vi "Turret_Aim.vi"(6 "View Button":bool, 7 "Left Trigger":dbl, 8 "Orange Limit Pressed":bool, 9 "Blue Limit Pressed":bool, 10 "Right Bumper":bool, 11 "Left Bumper":bool) -> ()   [LabVIEW 2020]
uses:
  <vilib>/Rock Robotics/WPI/ThirdParty/Phoenix-LabVIEW/Motor Controller/Controls/CTRE_Phoenix_MotorControl_ControlMode.ctl
  <vilib>/Rock Robotics/WPI/ThirdParty/Phoenix-LabVIEW/Motor Controller/Get/CTRE_Phoenix_MotorController_IntegratedSensorData_TalonFX.vi
  <vilib>/Rock Robotics/Network Tables/NT Read Number.vi
  <vilib>/addons/control/pid/pid.llb/PID (DBL).vi
  <vilib>/Rock Robotics/Network Tables/NT Write Number.vi
  <vilib>/addons/control/pid/NI_PID_pid.lvlib
panel:
  in  "Auto Center PID":T1={"proportional gain (Kc)"=-0.025, "integral time (Ti, min)"=0.0, "derivative time (Td, min)"=2e-05} {"derivative time (Td, min)" format="%.6f"; "integral time (Ti, min)" format="%.3f"; "proportional gain (Kc)" format="%.3f"}
  out "Ty":dbl
  out "Tx":dbl
  in  "Turret Auto Aim PID":T1={"proportional gain (Kc)"=-0.025, "integral time (Ti, min)"=0.0, "derivative time (Td, min)"=2e-05} {"derivative time (Td, min)" format="%.6f"; "integral time (Ti, min)" format="%.3f"; "proportional gain (Kc)" format="%.3f"}
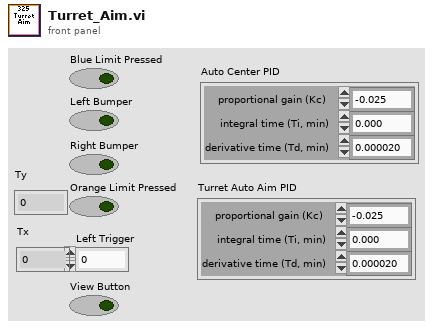
[diagram p1: front panel]
types:
  T1 = cluster{"proportional gain (Kc)":dbl, "integral time (Ti, min)":dbl, "derivative time (Td, min)":dbl}
  T2 = typedef "CTRE_Phoenix_MotorControl_ControlMode.ctl" = u16
  T3 = typedef "WPI_MotorControlDeviceRef.ctl" = cluster{"DeviceStatus":errorcluster, "Type":T4, "PWM":cluster{"PWM Channel":T5, "DeadBand":T6}, "CAN":cluster{"Device Number":u8, "SetOutput VI Ref":variant, "GetOutput VI Ref":variant, "Enable VI Ref":variant, "Disable VI Ref":variant, "Data":variant}, "Invert":bool, "DIO PWM":cluster{"PWM \"Enable\" Channel":T5, "DIOChannel":T7, "PWM Rate":dbl}}
  T4 = typedef "WPI_MotorControlType.ctl" = enum16{"PWM", "CAN", "DIO PWM"}
  T5 = typedef "FPGA_DIOPWMChannel.ctl" = enum8{"PWM 0", "PWM 1", "PWM 2", "PWM 3", "PWM 4", "PWM 5", "PWM 6", "PWM 7", "PWM 8", "PWM 9", "PWM MXP 0", "PWM MXP 1", "PWM MXP 2", "PWM MXP 3", "PWM MXP 4", "PWM MXP 5", "PWM MXP 6", "PWM MXP 7", "PWM MXP 8", "PWM MXP 9", "Invalid"}
  T6 = typedef "WPI_PWMDeadband.ctl" = cluster{"Name":string, "maxPositivePwm":i32, "minPositivePwm":i32, "centerPwm":i32, "maxNegativePwm":i32, "minNegativePwm":i32, "angularRange":u16}
  T7 = typedef "FPGA_DIOChannel.ctl" = enum8{"DIO 0", "DIO 1", "DIO 2", "DIO 3", "DIO 4", "DIO 5", "DIO 6", "DIO 7", "DIO 8", "DIO 9", "DIO MXP 0", "DIO MXP 1", "DIO MXP 2", "DIO MXP 3", "DIO MXP 4", "DIO MXP 5", "DIO MXP 6", "DIO MXP 7", "DIO MXP 8", "DIO MXP 9", "DIO MXP 10", "DIO MXP 11", "DIO MXP 12", "DIO MXP 13", "DIO MXP 14", "DIO MXP 15", "SPI Port CS1", "SPI Port CS2", "SPI Port CS3", "SPI Port MISO", "SPI Port MOSI", "Invalid"}
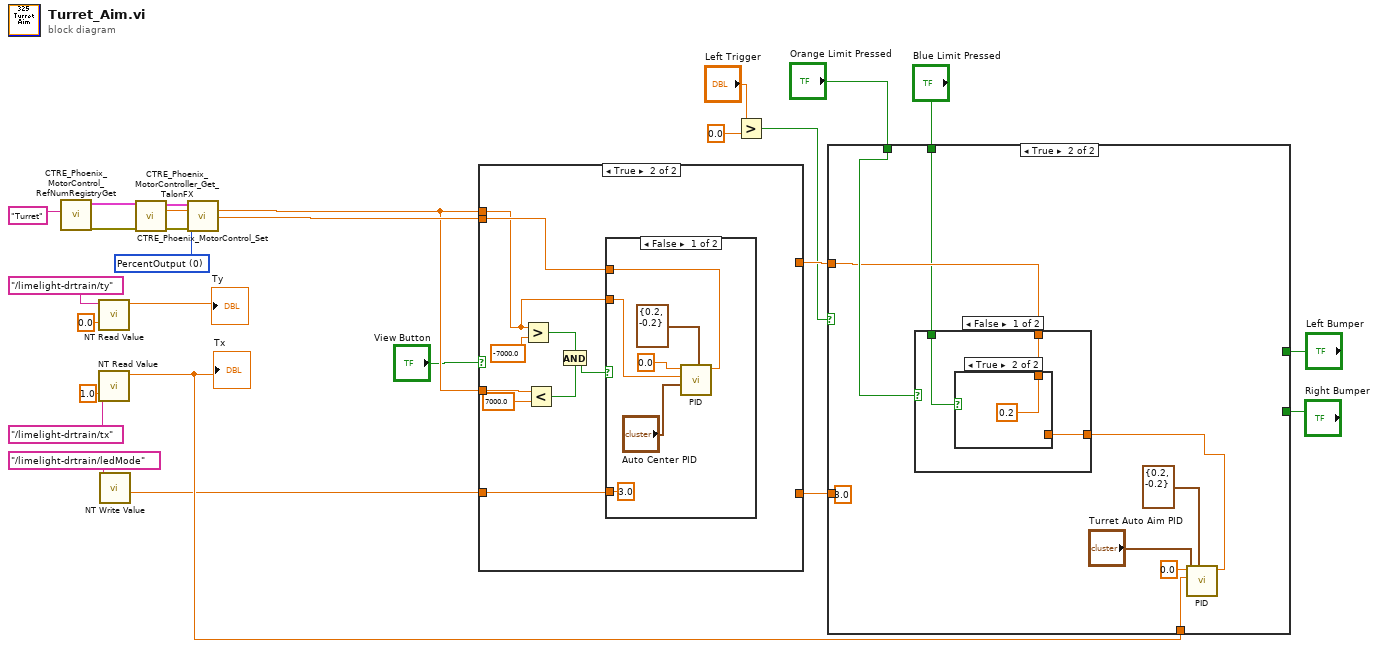
[diagram p0: block diagram]
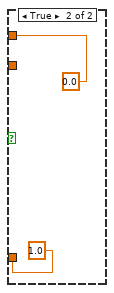
[diagram p3: hidden frame]
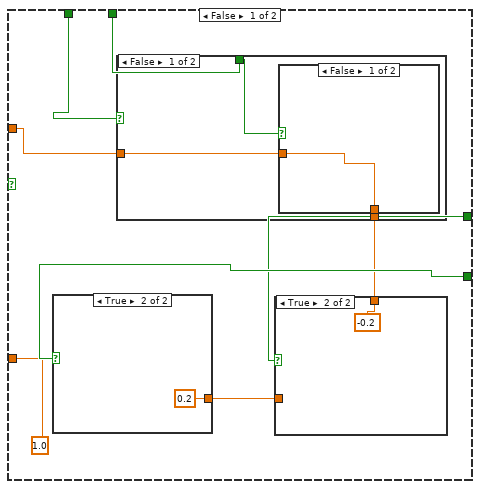
[diagram p4: hidden frame]
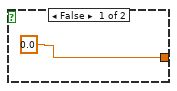
[diagram p6: hidden frame]
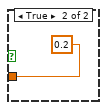
[diagram p7: hidden frame]
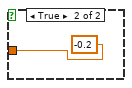
[diagram p8: hidden frame]
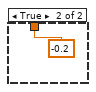
[diagram p10: hidden frame]
diagram:
  w25 = T2 0 items=["PercentOutput"=0, "Position"=1, "Velocity"=2, "Current"=3, "Follower"=5, "MotionProfile"=6, "MotionMagic"=7, "MotionProfileArc"=10, "Disabled"=15] ("Control Mode")
  n1 = call <vilib>:"CTRE_Phoenix_MotorControl_RefNumRegistryGet.vi"("refnum name"="Turret") -> ("error out"=w1:errorcluster, "PhoenixMotorControlDevRef"=w17:T3)  [unwired: 9 in]
  n2 = call-poly <vilib>:"NT Read Value.vi"("Default Value"=0.0, "Name"="/limelight-drtrain/ty") -> ("Numeric"=→"Ty":dbl)  [unwired: 8 in, 1 out]
  n3 = call-poly <vilib>:"NT Read Value.vi"("Default Value"=1.0, "Name"="/limelight-drtrain/tx") -> ("Numeric"=w6:dbl)  [unwired: 8 in, 1 out]
  "Tx" <- w6
  n4 = call-poly <vilib>:"CTRE_Phoenix_MotorController_Get_TalonFX.vi"("PhoenixMotorControlDevRef"=w17, "error in"=w1) -> ("PhoenixMotorControlDevRef"=w16:T3, "Position"=w4:dbl, "error out"=w15:errorcluster)  [unwired: 9 in, 2 out]
  n5 = Greater?(x="Left Trigger", y=0.0) -> (0:w5:bool)
  n6 = case shown="True" w5 {
    tunnel: [w28 w49] -> w12
    tunnel: "Orange Limit Pressed" -> [w34 w50]
    tunnel: "Blue Limit Pressed" -> [w33 w47]
    tunnel: "Right Bumper" -> [w32 _]
    tunnel: "Left Bumper" -> [w31 _]
    tunnel: [1.0 ("Numeric") 3.0 ("ledMode")] -> w13
    tunnel: w6 -> [_ w45]
    frame False {
      n7 = case shown="True" w32 {
        tunnel: [0.0 ("output") 0.2 ("output")] -> w30
        frame False {
        }
        frame True {
        }
      }
      n8 = case shown="True" w31 {
        tunnel: w30 -> [w35 _]
        tunnel: [w35 -0.2 ("output")] -> w29
        frame False {
        }
        frame True {
        }
      }
      n9 = case shown="False" w34 {
        tunnel: w33 -> [w41 _]
        tunnel: w29 -> [w40 _]
        tunnel: [w39 -0.2 ("output")] -> w28
        frame False {
          n10 = case shown="False" w41 {
            tunnel: w40 -> [w42 _]
            tunnel: [w42 0.2 ("output")] -> w39
            frame False {
            }
            frame True {
            }
          }
        }
        frame True {
        }
      }
    }
    frame True {
      n11 = call-poly <vilib>:"PID.vi"("output range"=cluster{"output high":dbl, "output low":dbl} {"output high"=0.2, "output low"=-0.2}, "PID gains"="Turret Auto Aim PID", "process variable"=w45, "setpoint"=0.0) -> ("output"=w48:dbl)  [unwired: 6 in, 1 out]
      n12 = case shown="False" w50 {
        tunnel: [w55 -0.2 ("output")] -> w49
        tunnel: w48 -> [w54 _]
        tunnel: w47 -> [w56 _]
        frame False {
          n13 = case shown="True" w56 {
            tunnel: [w57 0.2 ("output")] -> w55
            tunnel: w54 -> [w57 _]
            frame False {
            }
            frame True {
            }
          }
        }
        frame True {
        }
      }
    }
  }
  n14 = case shown="True" "View Button" {
    tunnel: w13 -> [w60 _]
    tunnel: w12 -> [w61 _]
    tunnel: [w61 w64] -> w14
    tunnel: w4 -> [_ w63]
    tunnel: w4 -> [_ w68]
    tunnel: [w60 w62] -> w2
    frame False {
    }
    frame True {
      n15 = Greater?(x=w63, y=-7000.0) -> (0:w70:bool)
      n16 = Less?(x=w68, y=7000.0) -> (x < y?=w69:bool)
      n17 = And(x=w70, y=w69) -> (x .and. y?=w67:bool)
      n18 = case shown="False" w67 {
        tunnel: [w72 0.0 ("output")] -> w64
        tunnel: w63 -> [w75 _]
        tunnel: [3.0 ("ledMode") 1.0 ("ledMode")] -> w62
        frame False {
          n19 = call-poly <vilib>:"PID.vi"("output range"=cluster{"output high":dbl, "output low":dbl} {"output high"=0.2, "output low"=-0.2}, "PID gains"="Auto Center PID", "process variable"=w75, "setpoint"=0.0) -> ("output"=w72:dbl)  [unwired: 6 in, 1 out]
        }
        frame True {
        }
      }
    }
  }
  n20 = call-poly <vilib>:"NT Write Value.vi"("Numeric"=w2, "Name"="/limelight-drtrain/ledMode") -> ()  [unwired: 9 in, 1 out]
  n21 = call <vilib>:"CTRE_Phoenix_MotorControl_Set.vi"("error in (no error)"=w15, "Output"=w14, "Control Mode"=w25, "PhoenixMotorControlDevRef"=w16) -> ()  [unwired: 6 in, 2 out]
